vi "Generate Dummy Digitizer Main Correction Text.vi"(11 "Digitizer identifications":string[](array[string])) -> (0 "Channels file names":string[](array[string]), 1 "Channels directories":string[](array[string]), 3 "main digitizer correction info file":string)   [LabVIEW 2020]
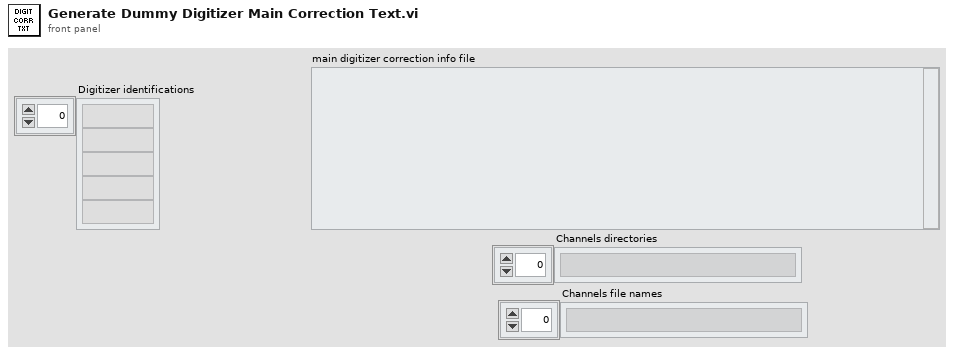
[diagram p1: front panel]
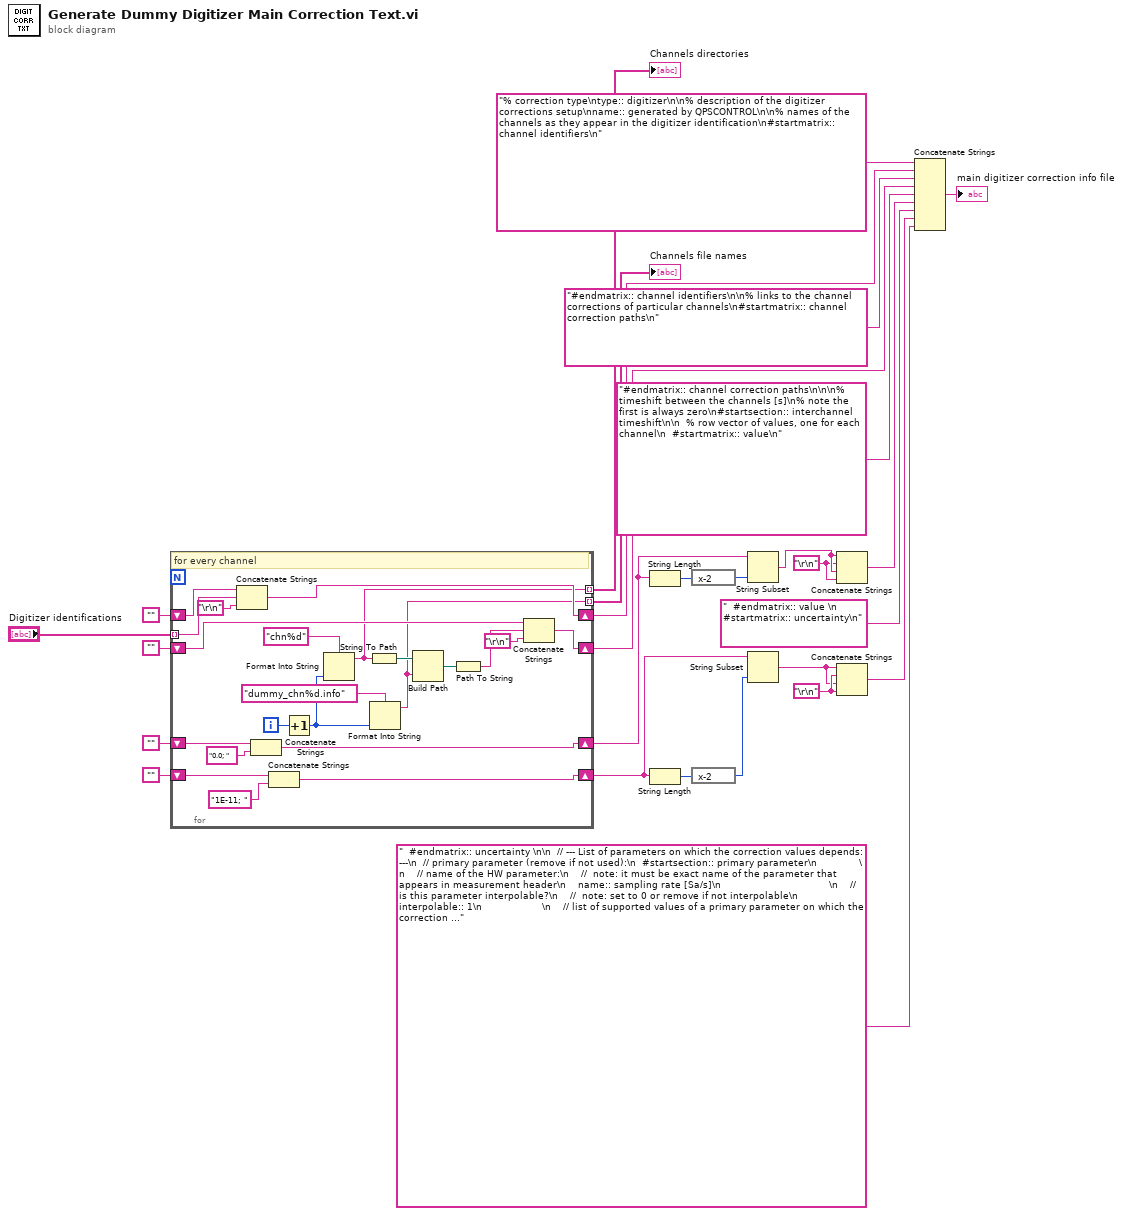
[diagram p0: block diagram]
diagram:
  w6 = "\r\n"
  w8 = "\r\n"
  n1 = for {
    tunnel: "Digitizer identifications" -> [w37] mode=indexing
    shift-right: [w48] -> w20
    shift-left: "" -> [w49]
    shift-right: [w44] -> w22
    shift-left: "" -> [w45]
    shift-right: [w42] -> w12
    shift-left: "" -> [w43]
    shift-right: [w40] -> w1
    shift-left: "" -> [w41]
    tunnel: [w29] -> w14 mode=indexing
    tunnel: [w28] -> w13 mode=indexing
    i -> [w36]
    # "for every channel"
    n2 = Concatenate Strings(w49, w37, "\r\n") -> (w48:string)
    n3 = Concatenate Strings(w43, "0.0; " ("format string")) -> (w42:string)
    n4 = Concatenate Strings(w41, "1E-11; " ("format string")) -> (w40:string)
    n5 = Increment(x=w36) -> (x+1=w34:i32)
    n6 = Format Into String(format string="chn%d", w34) -> (resulting string=w29:string)  [unwired: 2 in, 1 out]
    n7 = String To Path(string=w29) -> (path=w32:path)
    n8 = Format Into String(format string="dummy_chn%d.info", w34) -> (resulting string=w28:string)  [unwired: 2 in, 1 out]
    n9 = Build Path(base path=w32, name or relative path=w28) -> (appended path=w31:path)
    n10 = Path To String(path=w31) -> (string=w30:string)
    n11 = Concatenate Strings(w45, w30, "\r\n") -> (w44:string)
  }
  "Channels directories" <- w14
  "Channels file names" <- w13
  n12 = String Length(string=w12) -> (length=w10:i32)
  n13 = String Length(string=w1) -> (length=w4:i32)
  n14 = expression code="x-2"(w10) -> (w11:i32)
  n15 = expression code="x-2"(w4) -> (w3:i32)
  n16 = String Subset(string=w12, length (rest)=w11) -> (substring=w9:string)  [unwired: 1 in]
  n17 = String Subset(string=w1, length (rest)=w3) -> (substring=w5:string)  [unwired: 1 in]
  n18 = Concatenate Strings(w9, w8, w9, w8) -> (w7:string)
  n19 = Concatenate Strings(w5, w6, w5, w6) -> (w2:string)
  n20 = Concatenate Strings("% correction type\ntype:: digitizer\n\n% description of the digitizer corrections setup\nname:: generated by QPSCONTROL\n\n% names of the channels as they appear in the digitizer identification\n#startmatrix:: channel identifiers\n", w20, "#endmatrix:: channel identifiers\n\n% links to the channel corrections of particular channels\n#startmatrix:: channel correction paths\n", w22, "#endmatrix:: channel correction paths\n\n\n% timeshift between the channels [s]\n% note the first is always zero\n#startsection:: interchannel timeshift\n\n  % row vector of values, one for each channel\n  #startmatrix:: value\n", w7, "  #endmatrix:: value \n  #startmatrix:: uncertainty\n", w2, "  #endmatrix:: uncertainty \n\n  // --- List of parameters on which the correction values depends: ---\n  // primary parameter (remove if not used):\n  #startsection:: primary parameter\n              \n    // name of the HW parameter:\n    //  note: it must be exact name of the parameter that appears in measurement header\n    name:: sampling rate [Sa/s]\n                                    \n    // is this parameter interpolable?\n    //  note: set to 0 or remove if not interpolable\n    interpolable:: 1\n                    \n    // list of supported values of a primary parameter on which the correction depends:\n    //  eg.: range of the digitizer\n    #startmatrix:: value\n            1e1\n            1e7\n    #endmatrix:: value\n                \n  #endsection:: primary parameter\n\n#endsection:: interchannel timeshift") -> (→"main digitizer correction info file":string)
